vi "cm2nm_checkPairing.vi"(8 "Tab Control":T2(tab), 9 "CurrentSessionOut":T6[](array[typedef])=[{"MetaDataFile"=path "", "X"=-1.1, "Y"=0.0, "Group"=0, "Z"=0.0, "Rotation"=0.0, "Fiducial"=TRUE, "Magnification"=0.0, "Working_Distance"=0.0, "Notes"="", "Location Name/ID"="", "OtherRelatedDataFiles"=[], "Available"=FALSE}, {"MetaDataFile"=path "", "X"=0.0, "Y"=-1.0, "Group"=0, "Z"=0.0, "Rotation"=0.0, "Fiducial"=TRUE, "Magnification"=0.0, "Working_Distance"=0.0, "Notes"="", "Location Name/ID"="", "OtherRelatedDataFiles"=[], "Available"=FALSE}, {"MetaDataFile"=path "", "X"=0.0, "Y"=1.0, "Group"=0, "Z"=0.0, "Rotation"=0.0, "Fiducial"=TRUE, "Magnification"=0.0, "Working_Distance"=0.0, "Notes"="", "Location Name/ID"="", "OtherRelatedDataFiles"=[], "Available"=FALSE}, {"MetaDataFile"=path "", "X"=1.0, "Y"=0.0, "Group"=0, "Z"=0.0, "Rotation"=0.0, "Fiducial"=TRUE, "Magnification"=0.0, "Working_Distance"=0.0, "Notes"="", "Location Name/ID"="", "OtherRelatedDataFiles"=[], "Available"=FALSE}] {"Rotation" min=-37480660.29033894 max=37480660.27288565}, 10 "PairedFiducials":T4(array[cluster])=[{"X1"=1.1, "X2"=-1.1, "Y1"=0.0, "Y2"=0.0, "Z1"=0.0, "Z2"=0.0}, {"X1"=0.0, "X2"=0.0, "Y1"=1.0, "Y2"=-1.0, "Z1"=0.0, "Z2"=0.0}, {"X1"=0.0, "X2"=0.0, "Y1"=-1.0, "Y2"=1.0, "Z1"=0.0, "Z2"=0.0}, {"X1"=-1.0, "X2"=1.0, "Y1"=0.0, "Y2"=0.0, "Z1"=0.0, "Z2"=0.0}], 11 "Distances":dbl[](array[numeric])) -> (3 "Cancelled?":bool)   [LabVIEW 2010]
doc: "Use this template to create a dialog box with event handling."
uses:
  cm2nm_coordinate_information_v2.ctl
panel:
  in  "Cluster":T1
  in  "Manually Select Pairing":bool
  in  "Assign Reference\nName to Target":bool
  in  "Array":T3(array[cluster])
  out "Waveform Chart":dbl[](graph)
  out "load fiducial Names":bool
  in  "PairedFiducialNames":T5(array[cluster])
  in  "ReferenceSessionDataSet":T6[](array[typedef])=[{"MetaDataFile"=path "", "X"=-1.1, "Y"=0.0, "Group"=0, "Z"=0.0, "Rotation"=0.0, "Fiducial"=TRUE, "Magnification"=0.0, "Working_Distance"=0.0, "Notes"="", "Location Name/ID"="", "OtherRelatedDataFiles"=[], "Available"=FALSE}, {"MetaDataFile"=path "", "X"=0.0, "Y"=-1.0, "Group"=0, "Z"=0.0, "Rotation"=0.0, "Fiducial"=TRUE, "Magnification"=0.0, "Working_Distance"=0.0, "Notes"="", "Location Name/ID"="", "OtherRelatedDataFiles"=[], "Available"=FALSE}, {"MetaDataFile"=path "", "X"=0.0, "Y"=1.0, "Group"=0, "Z"=0.0, "Rotation"=0.0, "Fiducial"=TRUE, "Magnification"=0.0, "Working_Distance"=0.0, "Notes"="", "Location Name/ID"="", "OtherRelatedDataFiles"=[], "Available"=FALSE}, {"MetaDataFile"=path "", "X"=1.0, "Y"=0.0, "Group"=0, "Z"=0.0, "Rotation"=0.0, "Fiducial"=TRUE, "Magnification"=0.0, "Working_Distance"=0.0, "Notes"="", "Location Name/ID"="", "OtherRelatedDataFiles"=[], "Available"=FALSE}] {"Rotation" min=-37480660.29033894 max=37480660.27288565}
  in  "Cancel":bool
  in  "OK":bool
  # "Target Session Info"
  # "Reference Session Info"
  # "Not enabled yet\nnext version feature."
  # "Target Session Info"
  # "Reference Session Info"
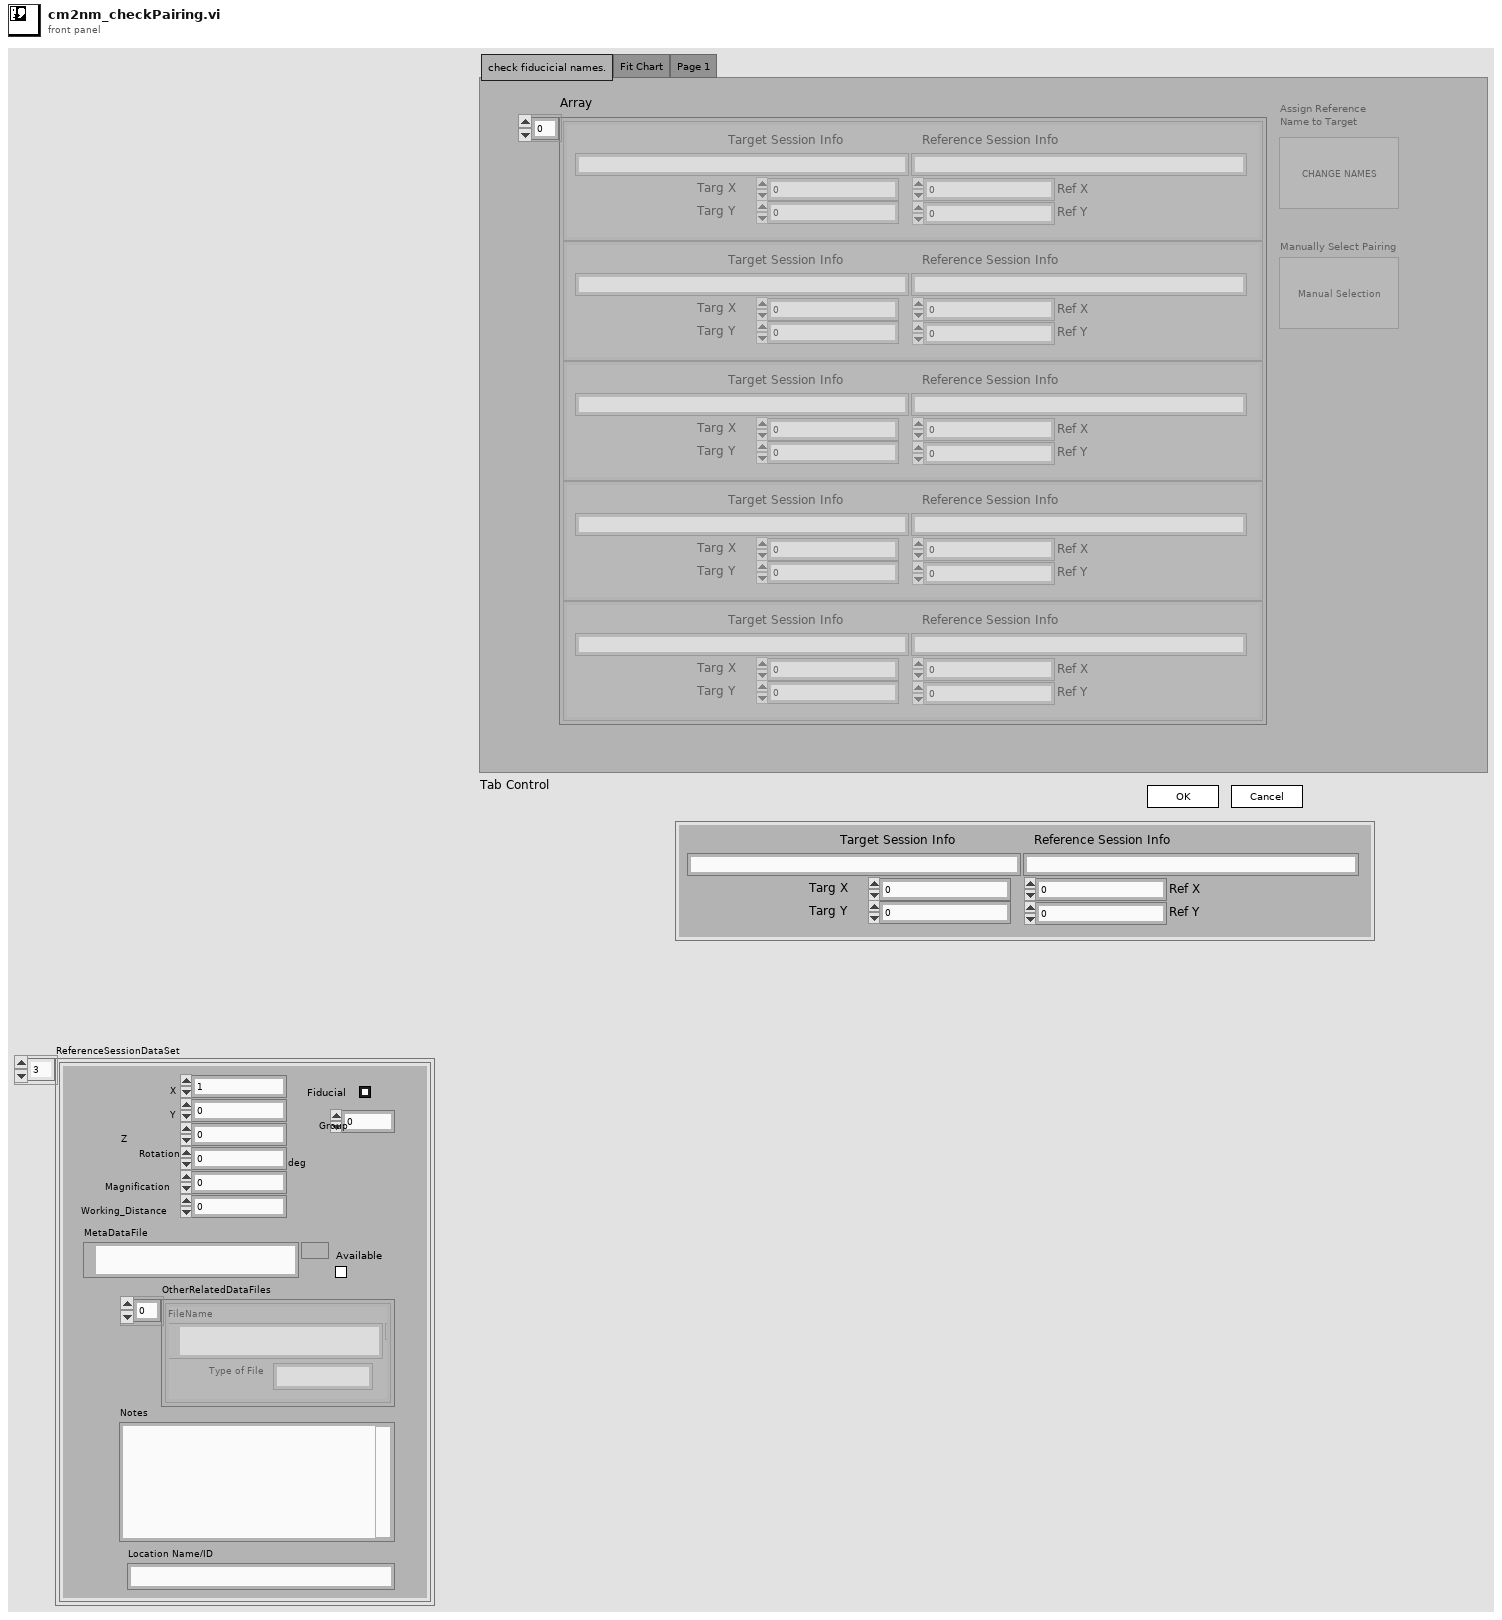
[diagram p1: front panel]
types:
  T1 = cluster{"Current Session Name":string, "Reference Session Name":string, "Targ X":dbl, "Targ Y":dbl, "Ref X":dbl, "Ref Y":dbl}
  T2 = enum32{"check fiducicial names.", "Fit Chart", "Page 1"}
  T3 = cluster{"Current Session Name":string, "Reference Session Name":string, "Targ X":dbl, "Targ Y":dbl, "Ref X":dbl, "Ref Y":dbl}[]
  T4 = cluster{"X1":dbl, "X2":dbl, "Y1":dbl, "Y2":dbl, "Z1":dbl, "Z2":dbl}[]
  T5 = cluster{"Location Name/ID":string, "Location Name/ID":string}[]
  T6 = typedef "cm2nm_coordinate_information_v2.ctl" = cluster{"MetaDataFile":path, "X":dbl, "Y":dbl, "Group":i32, "Z":dbl, "Rotation":dbl[unit], "Fiducial":bool, "Magnification":dbl, "Working_Distance":dbl, "Notes":string, "Location Name/ID":string, "OtherRelatedDataFiles":cluster{"Type of File":string, "FileName":path}[], "Available":bool}
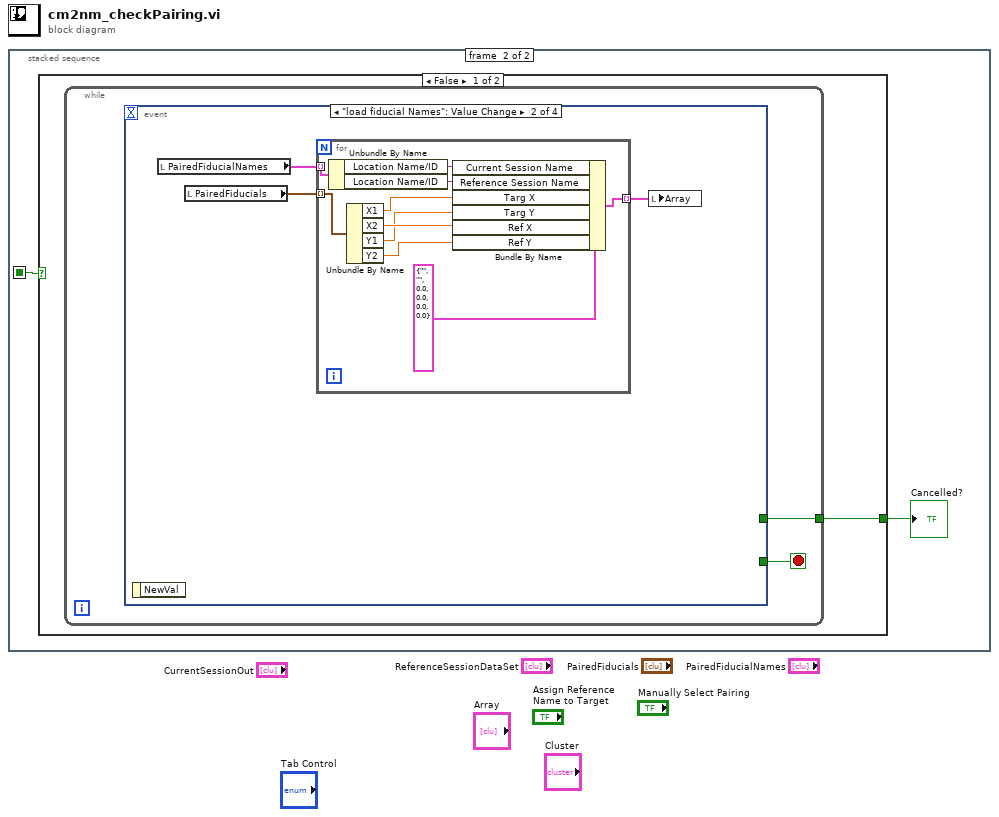
[diagram p0: block diagram]
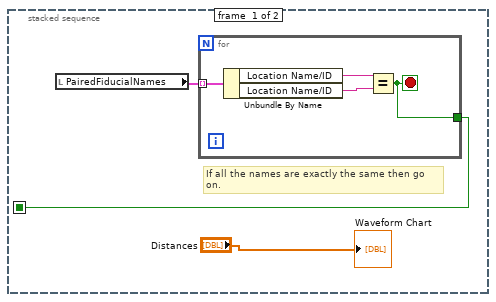
[diagram p2: hidden frame]
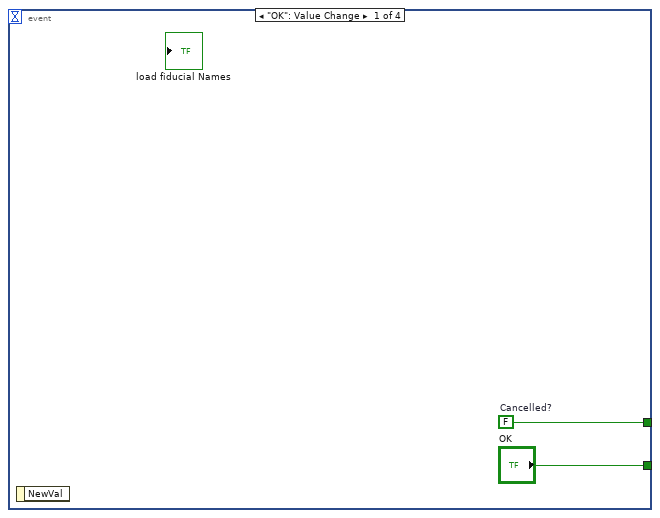
[diagram p3: hidden frame]
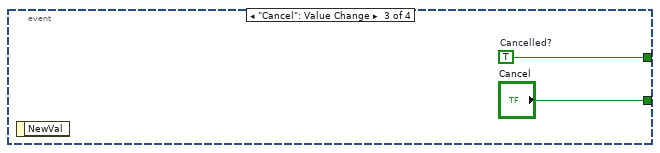
[diagram p4: hidden frame]
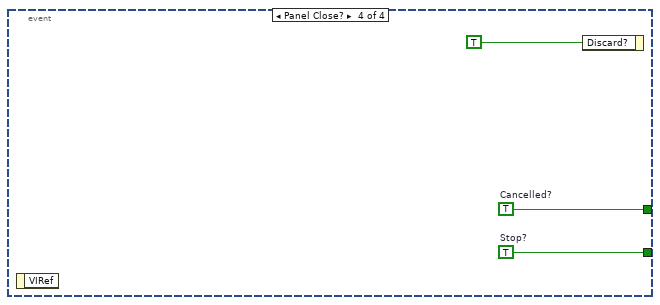
[diagram p5: hidden frame]
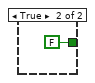
[diagram p6: hidden frame]
diagram:
  n1 = stacked-sequence {
    seq-local: [w2 _] -> [_ w8]
    frame #0 {
      # "If all the names are exactly the same then go\non."
      n2 = local read "PairedFiducialNames"() -> (w3:T5)
      n3 = for {
        tunnel: w3 -> [w7] mode=indexing
        tunnel: [w4] -> w2
        stop <- w4 stop-if-true
        n4 = Unbundle By Name(w7) -> ("Location Name/ID"=w6:string, "Location Name/ID"=w5:string)
        n5 = Equal?(x=w6, y=w5) -> (x = y?=w4:bool)
      }
      "Waveform Chart" <- "Distances"
    }
    frame #1 {
      n6 = case shown="False" w8 {
        tunnel: [w10 FALSE ("Cancelled?")] -> w9
        frame False {
          n7 = while {
            tunnel: [w11] -> w10
            stop <- w12 stop-if-true
            n8 = event shown="[1] \"load fiducial Names\": Value Change" {
              selector: _ -> [_ _ _ _]
              dyn-events: _ -> [_ _ _ _]
              timeout: _ -> [_ _ _ _]
              tunnel: ["OK" _ "Cancel" w31] -> w12
              tunnel: [w14 _ w29 w30] -> w11
              event "OK": Value Change {
                w14 = FALSE  # Cancelled?
                n9 = event-data() -> ()  [unwired: 1 in, 1 out]
              }
              event "load fiducial Names": Value Change {
                n10 = event-data() -> ()  [unwired: 1 in, 1 out]
                n11 = local read "PairedFiducialNames"() -> (w17:T5)
                n12 = local read "PairedFiducials"() -> (w16:T4)
                n13 = for {
                  tunnel: w17 -> [w27] mode=indexing
                  tunnel: w16 -> [w24] mode=indexing
                  tunnel: [w19] -> w15 mode=indexing
                  n14 = Unbundle By Name(w27) -> ("Location Name/ID"=w26:string, "Location Name/ID"=w25:string)
                  n15 = Unbundle By Name(w24) -> ("X1"=w23:dbl, "X2"=w22:dbl, "Y1"=w21:dbl, "Y2"=w20:dbl)
                  n16 = Bundle By Name(cluster=T1 {"Current Session Name"="", "Reference Session Name"="", "Targ X"=0.0, "Targ Y"=0.0, "Ref X"=0.0, "Ref Y"=0.0} ("Cluster"), "Current Session Name"=w26, "Reference Session Name"=w25, "Targ X"=w23, "Targ Y"=w21, "Ref X"=w22, "Ref Y"=w20) -> (w19:T1)
                }
                n17 = local write "Array"(w15) -> ()
              }
              event "Cancel": Value Change {
                w29 = TRUE  # Cancelled?
                n18 = event-data() -> ()  [unwired: 1 in, 1 out]
              }
              event Panel Close? {
                w30 = TRUE  # Cancelled?
                w31 = TRUE  # Stop?
                n19 = event-data() -> ()  [unwired: 1 in, 1 out]
                n20 = event-data("Discard?"=TRUE) -> ()  [unwired: 1 in, 1 out]
              }
            }
          }
        }
        frame True {
        }
      }
      "Cancelled?" <- w9
    }
  }
